vi "Vision Research Phantom Series PhFile PhGetSaveCineName.vi"(1 "CH in":u64, 5 "Error In (no error)":errorcluster) -> (15 "CH out":u64, 18 "Success":bool, 19 "Error Out":errorcluster)   [LabVIEW 2013, in "VRI.lvlib"]
doc: "PhFile.dll\n\nPhGetSaveCineName\nBOOL PhGetSaveCineName(CINEHANDLE CH);\n\nParameters Description\nCH(in,out) Handle of the cine to be saved.\nReturn TRUE – The operation has succeeded. The user ended the dialog with OK.\n FALSE – The operation has been canceled. The user ended the dialog with CANCEL.\nComments This function displays a dialog box for saving a cine file. The user can either select \n an existing file to be overwritten or create a new file.\n All the information about the user choices is stored in the cine handle.\n\nWritten by:\nBLOOMY CONTROLS, INC\nWINDSOR, CT 06095, USA\n860-298-9925\nwww.bloomy.com\nV1.0.0\nMay, 2004"
uses:
  VRI.lvlib
  Phantom DLLs/PhFile.dll
panel:
  # "For instructions on the use of this VI, press Ctrl+H to display the help window and move the mouse over the icon, controls, and indicators"
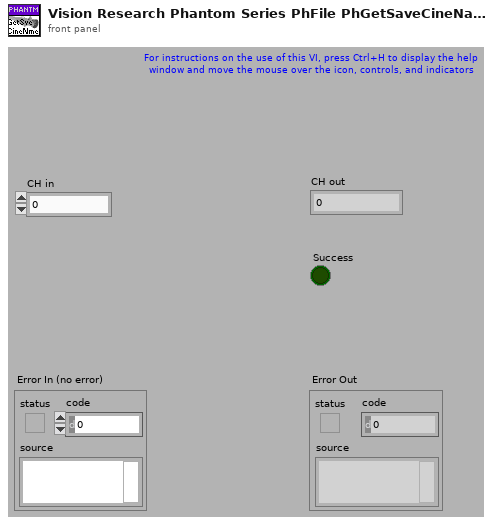
[diagram p1: front panel]
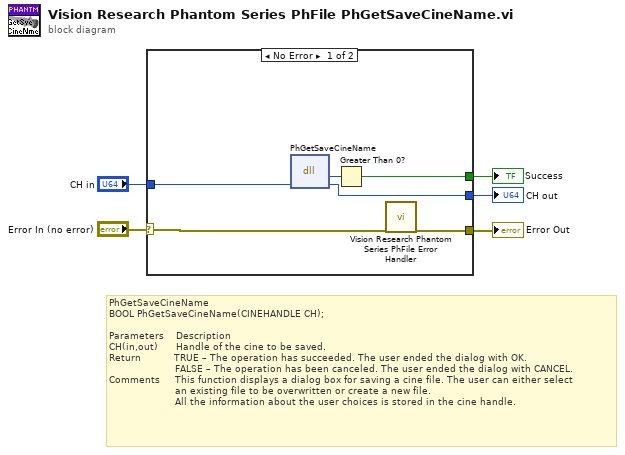
[diagram p0: block diagram]
diagram:
  # "PhGetSaveCineName\nBOOL PhGetSaveCineName(CINEHANDLE CH);\n\nParameters    Description\nCH(in,out)      Handle of the cine to be saved.\nReturn           TRUE – The operation has succeeded. The user ended the dialog with OK.\n                      FALSE – The operation has been canceled. The user ended the dialog with CANCEL.\nComments     This function displays a dialog box for saving a cine file. The user can either select \n                      an existing file to be overwritten or create a new file.\n                      All the information about the user choices is stored in the cine handle."
  n1 = case shown="No Error" "Error In (no error)" {
    selector: "Error In (no error)" -> [w11 w13]
    tunnel: [w10 w13] -> w4
    tunnel: [w9 _] -> w3
    tunnel: [w8 w12] -> w2
    tunnel: "CH in" -> [w7 w12]
    frame No Error {
      n2 = dll-call lib="C:/Projects/SDK/32-bit/Vision Research Phantom Series Labview Driver/Phantom DLLs/PhFile.dll" fn="PhGetSaveCineName"("CH"=w7) -> ("return type"=w6:i32, "CH"=w8:u64)  [unwired: 3 in, 2 out]
      n3 = Greater Than 0?(x=w6) -> (x > 0?=w9:bool)
      n4 = call "Vision Research Phantom Series PhFile Error Handler.vi"("Error In (no error)"=w11) -> ("Error Out"=w10:errorcluster)  [unwired: 1 in, 17 out]
    }
    frame Error {
    }
  }
  "Error Out" <- w4
  "Success" <- w3
  "CH out" <- w2
